vi "Complicated Function Generator.vi"(0 "frequency":dbl=10.0 format="%0.2p", 1 "signal type":T2(ring), 3 "offset":dbl format="%0.2p", 5 "amplitude":dbl=4.0 format="%0.2p", 7 "samples":dbl=1000.0 format="%0.2p", 9 "bufsize":dbl=1000.0 format="%#.2p", 11 "error in (no error)":errorcluster, 12 "Chans":u32, 14 "Tab Control":T1(ring)) -> (4 "Wave out":waveform(dbl), 6 "WfmArray":waveform(dbl)[](array[waveform]), 8 "DblArray":dbl[][](array[numeric]), 10 "DBL Out":dbl[](array[numeric]), 13 "Sync":bool, 15 "error out":errorcluster)   [LabVIEW 2010]
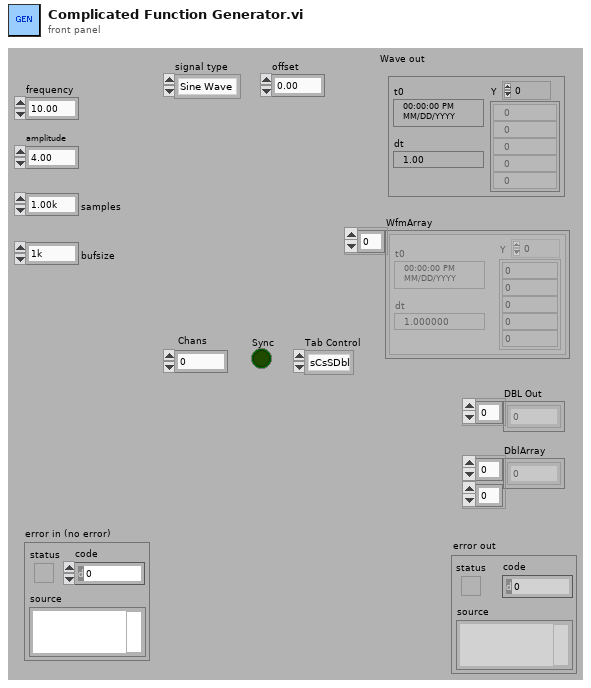
[diagram p1: front panel]
types:
  T1 = enum32{"sCsSDbl", "sCsSWfm", "sCnS1D", "sCnSWfm", "nCsSDbl", "nCsSWfm", "nCnS2D", "nCnS1DWfm", "2DI16", "2DI32", "2DU16", "2DU32"}
  T2 = enum16{"Sine Wave", "Triangle Wave", "Square Wave", "Sawtooth Wave"}
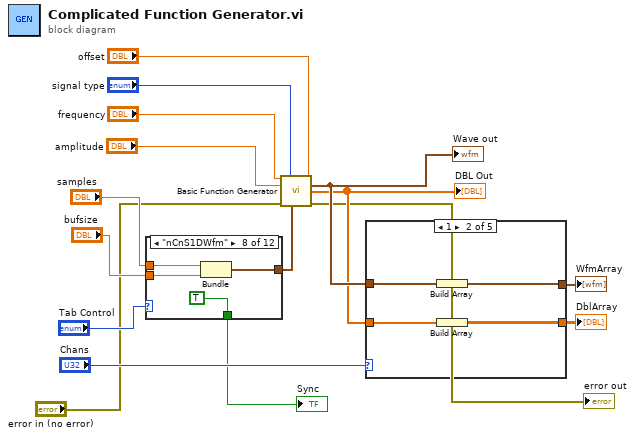
[diagram p0: block diagram]
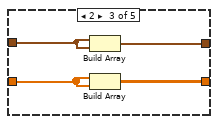
[diagram p3: hidden frame]
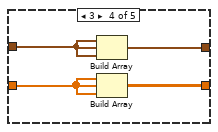
[diagram p4: hidden frame]
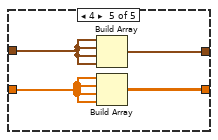
[diagram p5: hidden frame]
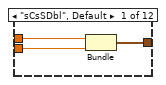
[diagram p6: hidden frame]
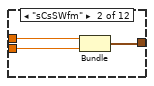
[diagram p7: hidden frame]
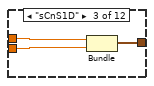
[diagram p8: hidden frame]
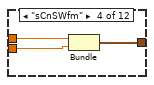
[diagram p9: hidden frame]
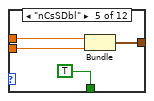
[diagram p10: hidden frame]
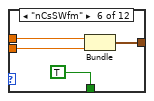
[diagram p11: hidden frame]
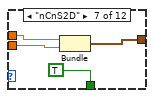
[diagram p12: hidden frame]
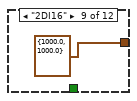
[diagram p13: hidden frame]
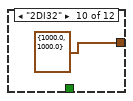
[diagram p14: hidden frame]
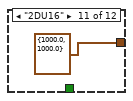
[diagram p15: hidden frame]
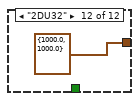
[diagram p16: hidden frame]
diagram:
  n1 = case shown="\"nCnS1DWfm\"" "Tab Control" {
    tunnel: [w17 w20 w25 w27 w32 w36 w38 w42 cluster{"samples":dbl, "bufsize":dbl} {"samples"=1000.0, "bufsize"=1000.0} cluster{"samples":dbl, "bufsize":dbl} {"samples"=1000.0, "bufsize"=1000.0} cluster{"samples":dbl, "bufsize":dbl} {"samples"=1000.0, "bufsize"=1000.0} cluster{"samples":dbl, "bufsize":dbl} {"samples"=1000.0, "bufsize"=1000.0}] -> w13
    tunnel: "samples" -> [w19 w22 w24 w28 w31 w35 w40 w44 _ _ _ _]
    tunnel: "bufsize" -> [w18 w21 w23 w26 w30 w34 w39 w43 _ _ _ _]
    tunnel: [_ _ _ _ TRUE TRUE TRUE TRUE _ _ _ _] -> w1
    frame "sCsSDbl", Default {
      n2 = Bundle("samples"=w19, "bufsize"=w18) -> (w17:cluster{"samples":dbl, "bufsize":dbl})  [unwired: 1 in]
    }
    frame "sCsSWfm" {
      n3 = Bundle("samples"=w22, "bufsize"=w21) -> (w20:cluster{"samples":dbl, "bufsize":dbl})  [unwired: 1 in]
    }
    frame "sCnS1D" {
      n4 = Bundle("samples"=w24, "bufsize"=w23) -> (w25:cluster{"samples":dbl, "bufsize":dbl})  [unwired: 1 in]
    }
    frame "sCnSWfm" {
      n5 = Bundle("samples"=w28, "bufsize"=w26) -> (w27:cluster{"samples":dbl, "bufsize":dbl})  [unwired: 1 in]
    }
    frame "nCsSDbl" {
      n6 = Bundle("samples"=w31, "bufsize"=w30) -> (w32:cluster{"samples":dbl, "bufsize":dbl})  [unwired: 1 in]
    }
    frame "nCsSWfm" {
      n7 = Bundle("samples"=w35, "bufsize"=w34) -> (w36:cluster{"samples":dbl, "bufsize":dbl})  [unwired: 1 in]
    }
    frame "nCnS2D" {
      n8 = Bundle("samples"=w40, "bufsize"=w39) -> (w38:cluster{"samples":dbl, "bufsize":dbl})  [unwired: 1 in]
    }
    frame "nCnS1DWfm" {
      n9 = Bundle("samples"=w44, "bufsize"=w43) -> (w42:cluster{"samples":dbl, "bufsize":dbl})  [unwired: 1 in]
    }
    frame "2DI16" {
    }
    frame "2DI32" {
    }
    frame "2DU16" {
    }
    frame "2DU32" {
    }
  }
  "Sync" <- w1
  n10 = call "Basic Function Generator.vi"("frequency"="frequency", "signal type"="signal type", "offset"="offset", "amplitude"="amplitude", "error in (no error)"="error in (no error)", "sampling info"=w13) -> ("signal out"=w8:waveform(dbl), "DBL Out"=w7:dbl[], "error out"=→"error out":errorcluster)  [unwired: 6 in, 1 out]
  "Wave out" <- w8
  "DBL Out" <- w7
  n11 = case shown="1" "Chans" {
    tunnel: w8 -> [_ w52 w56 w60 w62]
    tunnel: [_ w51 w54 w57 w63] -> w6
    tunnel: w7 -> [_ w50 w55 w59 w61]
    tunnel: [_ w49 w53 w58 w64] -> w5
    frame 0, Default {
    }
    frame 1 {
      n12 = Build Array(w52) -> (w51:waveform(dbl)[])
      n13 = Build Array(w50) -> (w49:dbl[][])
    }
    frame 2 {
      n14 = Build Array(w56, w56) -> (w54:waveform(dbl)[])
      n15 = Build Array(w55, w55) -> (w53:dbl[][])
    }
    frame 3 {
      n16 = Build Array(w60, w60, w60) -> (w57:waveform(dbl)[])
      n17 = Build Array(w59, w59, w59) -> (w58:dbl[][])
    }
    frame 4 {
      n18 = Build Array(w62, w62, w62, w62) -> (w63:waveform(dbl)[])
      n19 = Build Array(w61, w61, w61, w61) -> (w64:dbl[][])
    }
  }
  "WfmArray" <- w6
  "DblArray" <- w5
